vi "Test BMS communication.vi"() -> ()   [LabVIEW 2016]
uses:
  Program Files (x86)/National Instruments/LabVIEW 2016/examples/robotics/EPOS2 CANOpen Driver/Low Level VIs/Typedefs/FPGA CAN Frame Cluster.ctl
  Dashboard Control.ctl
  <vilib>/Utility/miscctls.llb/LVRowAndColumnUnsignedTypeDef.ctl
  <vilib>/Platform/TimedLoop/XDataNode/timing_clust.ctl
  <vilib>/Platform/TimedLoop/XDataNode/nitl_modes.ctl
  <vilib>/Platform/TimedLoop/XDataNode/wakeup.ctl
  RT/Read All CAN.vi
  <vilib>/Platform/TimedLoop/XDataNode/XDataNode.xnode
  <vilib>/Platform/TimedLoop/XDataNode/XDNodeRunTimeDep.lvlib
panel:
  in  "Tab Control":enum32{"Play!", "Debugg"}(tab)
  in  "Dashboard Control":T1 {"High Voltage" scale=0.0..255.0; "Low Voltage" scale=0.0..255.0}
  out "Tractive system activation":bool
  out "Ready to drive":bool
  in  "CAN Frame":T2={"Timestamp"=0, "Identifier"=0, "Type"=0, "InfoA"=0, "InfoB"=0, "DataLength"=0, "Data"=[0, 0, 0, 0, 0, 0, 0, 0]} {"Data" format="%.0x"; "DataLength" format="%.0x"; "InfoB" format="%.0x"; "InfoA" format="%.0x"; "Type" format="%.0x"; "Identifier" format="%.0x"; "Timestamp" format="%.0x"}
  in  "Send once":bool
  in  "Send cont.":bool
  in  "Stop":bool
  out "Error Out":errorcluster
  out "CAN Frame Out":T2 {"Data" format="%.0x"; "DataLength" format="%.0x"; "InfoB" format="%.0x"; "InfoA" format="%.0x"; "Type" format="%.0x"; "Identifier" format="%.0x"; "Timestamp" format="%.0x"}
  in  "Clear list":bool
  out "Multicolumn Listbox":i32(listbox)
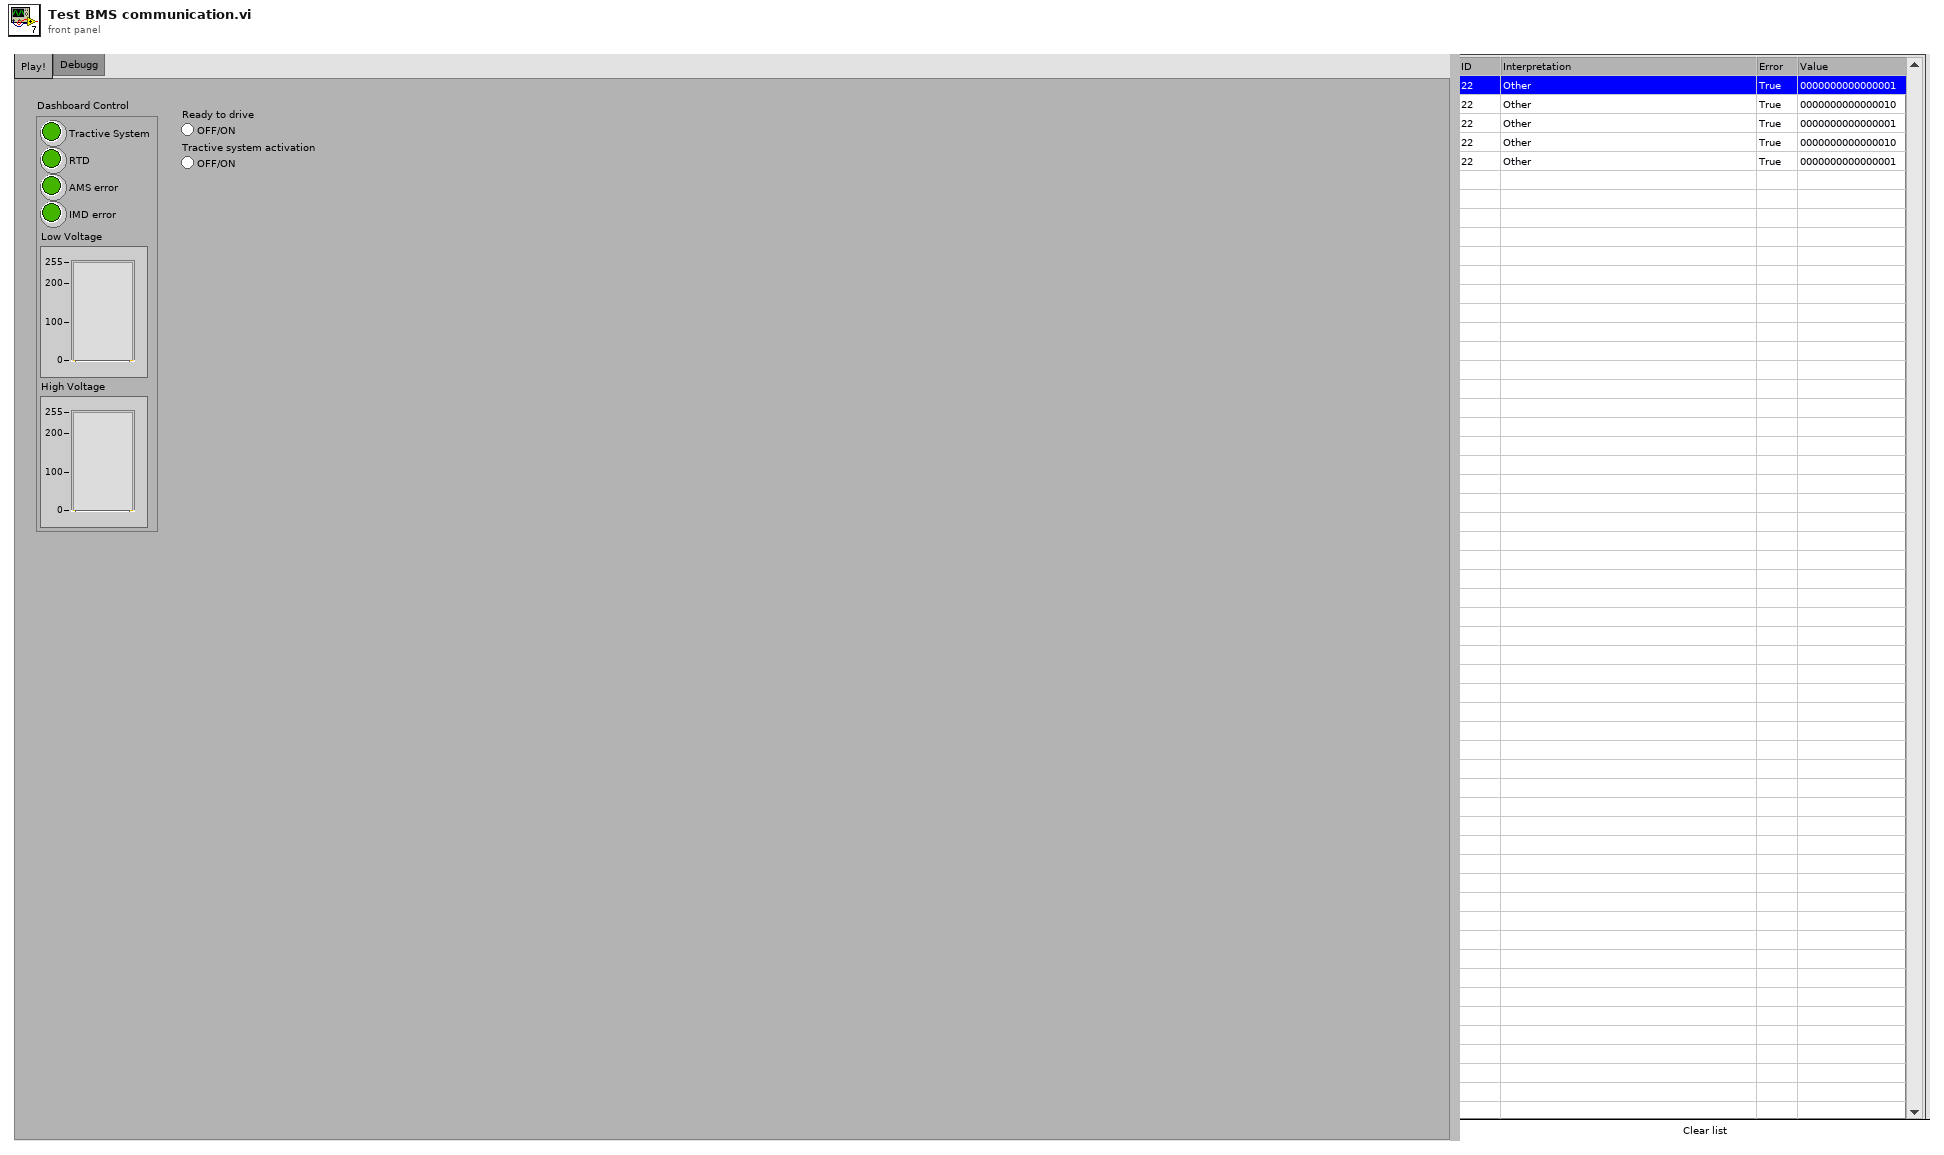
[diagram p1: front panel]
types:
  T1 = typedef "Dashboard Control.ctl" = cluster{"Tractive System":bool, "RTD":bool, "AMS error":bool, "IMD error":bool, "Low Voltage":dbl, "High Voltage":dbl}
  T2 = typedef "FPGA CAN Frame Cluster.ctl" = cluster{"Timestamp":u64, "Identifier":u32, "Type":u8, "InfoA":u8, "InfoB":u8, "DataLength":u8, "Data":u8[]}
  T3 = cluster{"Message":string, "ID":u16, "Error":bool}[]
  T4 = typedef "LVRowAndColumnUnsignedTypeDef.ctl" = cluster{"Row":u32, "Column":u32}
  T5 = typedef "XDNodeRunTimeDep.lvlib/timing_clust.ctl" = cluster{"Expected End [f-1]":u64, "Actual End [f-1]":u64, "Finished Late? [f-1]":bool, "Expected End [i-1]":u64, "Actual End [i-1]":u64, "Finished Late? [i-1]":bool, "Expected Start [i]":u64, "Actual Start [i]":u64, "Expected Start [f]":u64, "Actual Start [f]":u64, "Source Name":string, "Structure Name":string, "Period":i64, "Deadline":i64, "Offset":i64, "Start":i64, "Priority":i32, "Timeout":i32, "Mode":T6, "Wakeup Reason":T7, "Error":errorcluster, "Source Type":string, "Secondary Source Type":string, "Global End Time":u64, "Global Start Time":u64, "Frame Duration":u64, "Iteration Duration":u64, "Assigned CPU":i32, "I/O Scan Engine Mode":u32}
  T6 = typedef "XDNodeRunTimeDep.lvlib/nitl_modes.ctl" = enum32{"No Change", "Process missed periods, maintain original phase", "Discard missed periods, maintain original phase", "Process missed periods, ignore original phase", "Discard missed periods, ignore original phase"}
  T7 = typedef "XDNodeRunTimeDep.lvlib/wakeup.ctl" = enum32{"Normal", "Aborted", "Asynchronous wakeup", "Timing source error", "Timed loop error", "Timeout"}
  T8 = typedef "CAN Refnum.ctl" = refnum<k1>
  T9 = cluster{"Boolean array[0]":bool, "Boolean array[1]":bool, "Boolean array[2]":bool, "Boolean array[3]":bool, "Boolean array[4]":bool, "Boolean array[5]":bool, "Boolean array[6]":bool, "Boolean array[7]":bool, "Boolean array[8]":bool}
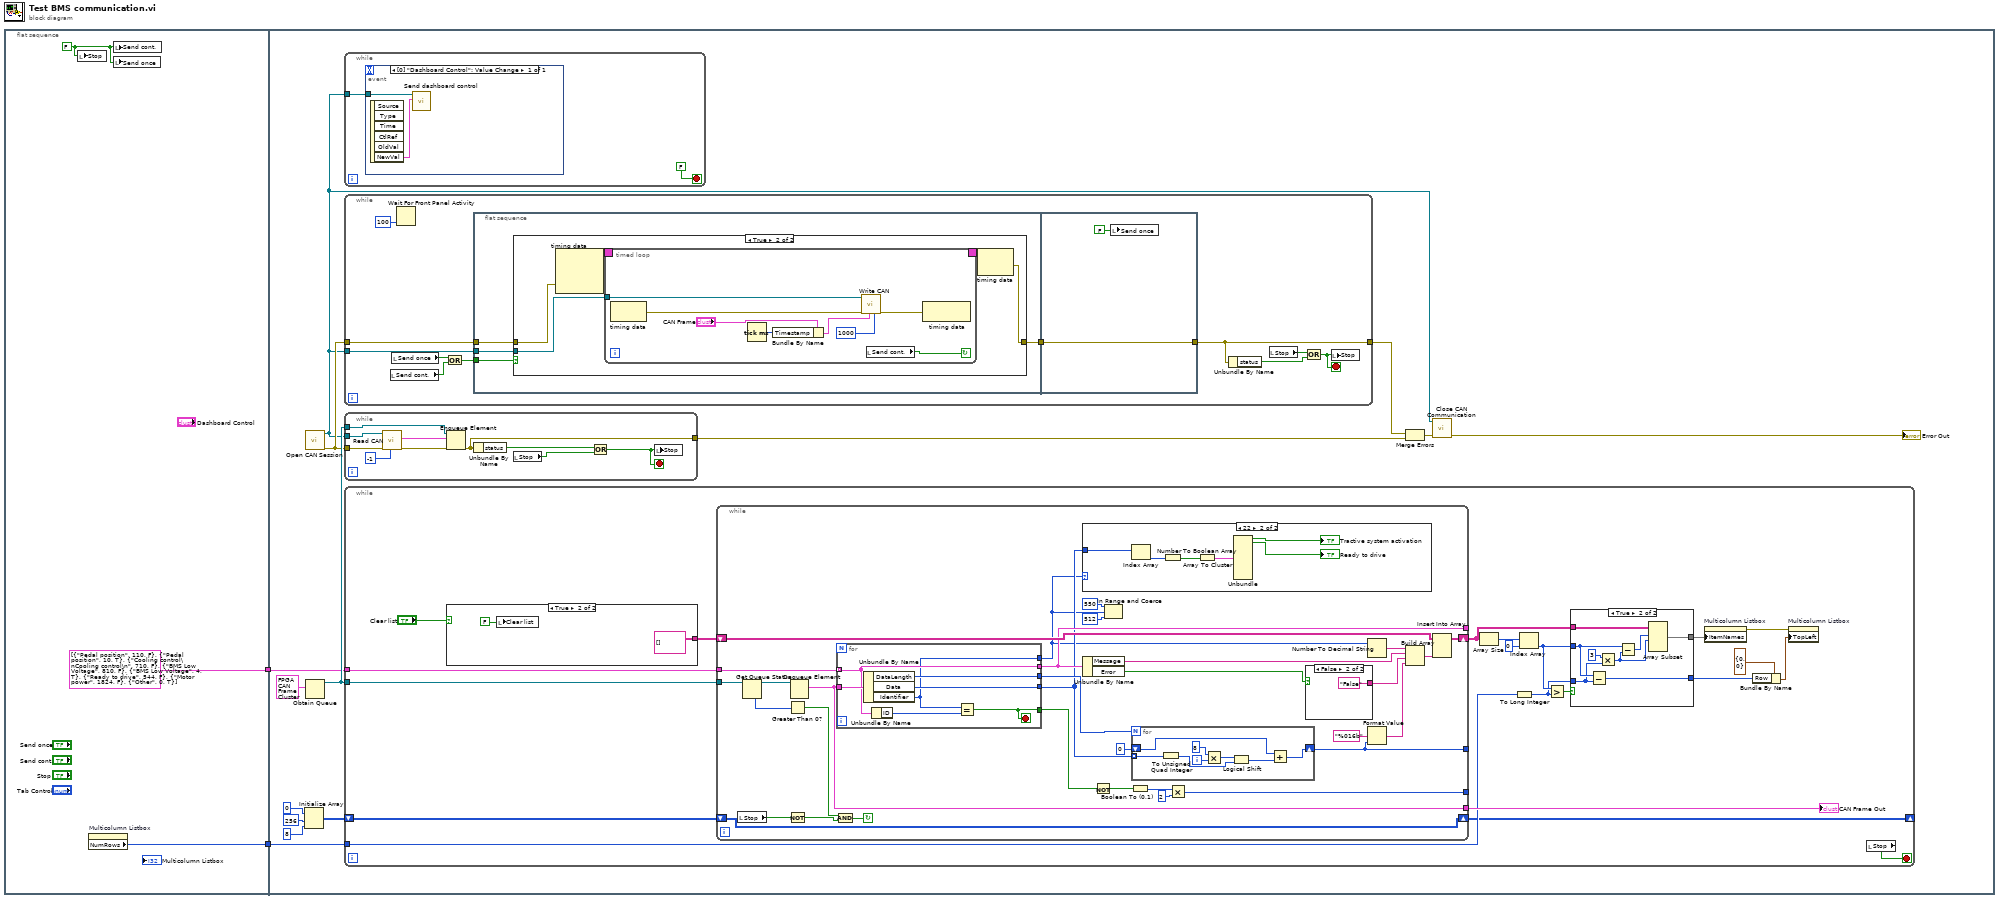
[diagram p0: block diagram]
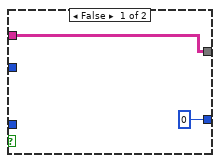
[diagram p2: hidden frame]
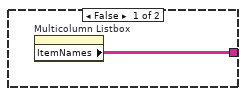
[diagram p3: hidden frame]
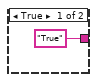
[diagram p5: hidden frame]
diagram:
  n1 = flat-sequence {
    tunnel: [w4] -> w2
    tunnel: [T3 [{"Message"="Pedal position", "ID"=110, "Error"=FALSE}, {"Message"="Pedal position", "ID"=10, "Error"=TRUE}, {"Message"="Cooling control\nCooling control\n", "ID"=710, "Error"=FALSE}, {"Message"="BMS Low Voltage", "ID"=810, "Error"=FALSE}, {"Message"="BMS Low Voltage", "ID"=4, "Error"=TRUE}, {"Message"="Ready to drive", "ID"=544, "Error"=FALSE}, {"Message"="Motor power", "ID"=1824, "Error"=FALSE}, {"Message"="Other", "ID"=0, "Error"=TRUE}] ("Messages")] -> w1
    tunnel: w2 -> [w14]
    tunnel: w1 -> [w13]
    frame #0 {
      w5 = FALSE
      n2 = local write "Stop"(w5) -> ()
      n3 = property on="Multicolumn Listbox" class="MCListbox (strict)"() -> ("NumRows"=w4:u32)  [unwired: 2 in, 2 out]
      n4 = local write "Send cont."(w5) -> ()
      n5 = local write "Send once"(w5) -> ()
    }
    frame #1 {
      n6 = Initialize Array(u8 0 ("element"), 256 ("dimension size"), 8 ("dimension size")) -> (w9:u8[][])
      n7 = call "Open CAN Session.vi"() -> ("error out"=w7:errorcluster, "CAN Session"=w6:T8)  [unwired: 10 in]
      n8 = Obtain Queue(element data type=T2 {"Timestamp"=0, "Identifier"=0, "Type"=0, "InfoA"=0, "InfoB"=0, "DataLength"=0, "Data"=[0, 0, 0, 0, 0, 0, 0, 0]} ("CAN Frame Out")) -> (queue out=w16:refnum<queue>)  [unwired: 4 in, 2 out]
      n9 = while {
        tunnel: w6 -> [w21]
        stop <- FALSE stop-if-true
        n10 = event shown="[0] \"Dashboard Control\": Value Change" {
          selector: _ -> [_]
          dyn-events: _ -> [_]
          timeout: _ -> [_]
          tunnel: w21 -> [w22]
          event Value Change {
            n11 = event-data() -> ("NewVal"=w23:T1)  [unwired: 1 in, 5 out]
            n12 = call "Send dashboard control.vi"("Dashboard Control"=w23, "CAN Session In"=w22) -> ()  [unwired: 8 in, 2 out]
          }
        }
      }
      n13 = while {
        tunnel: w7 -> [w132]
        tunnel: w6 -> [w131]
        tunnel: [w127] -> w18
        stop <- w123 stop-if-true
        n14 = local read "Send cont."() -> (w129:bool)
        n15 = local read "Send once"() -> (w128:bool)
        n16 = Wait For Front Panel Activity(1:100 ("timeout ms (-1 never timeout)")) -> ()  [unwired: 2 in, 1 out]
        n17 = Or(x=w128, y=w129) -> (x .or. y?=w130:bool)
        n18 = flat-sequence {
          tunnel: w132 -> [w136]
          tunnel: w131 -> [w135]
          tunnel: w130 -> [w134]
          tunnel: [w133] -> w122
          tunnel: [w162] -> w127
          tunnel: w122 -> [w162]
          frame #0 {
            n19 = case shown="True" w134 {
              tunnel: w136 -> [w137 w139]
              tunnel: w135 -> [_ w140]
              tunnel: [w137 w138] -> w133
              frame False {
              }
              frame True {
                n20 = node-c288(w139) -> (w142:T5)  [unwired: 2 in]
                n21 = timed-loop {
                  timing: w142 -> [_]
                  timing-out: [_] -> w141
                  tunnel: w140 -> [w150]
                  stop <- w147 continue-if-true
                  n22 = node-c288() -> (w149:errorcluster)  [unwired: 1 in]
                  n23 = Tick Count (ms)() -> (millisecond timer value=w143:u32)
                  n24 = Bundle By Name(cluster="CAN Frame", "Timestamp"=w143) -> (w144:T2)
                  n25 = call "Write CAN.vi"("timeout"=1000, "CAN Frame"=w144, "error in"=w149, "CAN Session In"=w150) -> ("error out"=w148:errorcluster)  [unwired: 6 in, 1 out]
                  n26 = local read "Send cont."() -> (w147:bool)
                  n27 = node-c288(w148) -> ()  [unwired: 1 out]
                }
                n28 = node-c288(w141) -> (w138:errorcluster)
              }
            }
          }
          frame #1 {
            n29 = local write "Send once"(FALSE) -> ()
          }
        }
        n30 = Unbundle By Name(w127) -> ("status"=w124:bool)
        n31 = local read "Stop"() -> (w125:bool)
        n32 = Or(x=w125, y=w124) -> (x .or. y?=w123:bool)
        n33 = local write "Stop"(w123) -> ()
      }
      n34 = while {
        tunnel: w7 -> [w113]
        tunnel: w6 -> [w112]
        tunnel: w16 -> [w119]
        tunnel: [w117] -> w15
        stop <- w120 stop-if-true
        n35 = call-poly "Read CAN.vi"("timeout in ms (-1)"=-1, "error in"=w113, "CAN Session In"=w112) -> ("error out"=w115:errorcluster, "CAN Frame Out"=w116:T2)  [unwired: 6 in, 1 out]
        n36 = Enqueue Element(queue=w119, element=w116, error in (no error)=w115) -> (error out=w117:errorcluster)  [unwired: 1 in, 2 out]
        n37 = Unbundle By Name(w117) -> ("status"=w118:bool)
        n38 = local read "Stop"() -> (w121:bool)
        n39 = Or(x=w118, y=w121) -> (x .or. y?=w120:bool)
        n40 = local write "Stop"(w120) -> ()
      }
      n41 = while {
        tunnel: w16 -> [w43]
        tunnel: w14 -> [w37]
        tunnel: w13 -> [w36]
        shift-right: [w24] -> _
        shift-left: w9 -> [w25]
        stop <- w41 stop-if-true
        n42 = case shown="True" "Clear list" {
          tunnel: [w54 string[][] [] ("Item Names")] -> w34
          frame False {
            n43 = property on="Multicolumn Listbox" class="MCListbox (strict)"() -> ("ItemNames"=w54:string[][])  [unwired: 2 in, 2 out]
          }
          frame True {
            n44 = local write "Clear list"(FALSE) -> ()
          }
        }
        n45 = while {
          tunnel: w43 -> [w86]
          tunnel: [w71] -> _
          tunnel: [w63] -> _
          tunnel: [w70] -> w42
          tunnel: [w69] -> _
          shift-right: [w72] -> w30
          shift-left: w34 -> [w73]
          tunnel: w36 -> [w68]
          shift-right: [w59] -> w24
          shift-left: w25 -> [w59]
          stop <- w64 continue-if-true
          n46 = local read "Stop"() -> (w67:bool)
          n47 = Get Queue Status(queue=w86) -> (queue out=w87:refnum<queue>, # elements in queue=w88:i32)  [unwired: 2 in, 6 out]
          n48 = Greater Than 0?(x=w88) -> (x > 0?=w65:bool)
          n49 = Not(x=w67) -> (.not. x?=w66:bool)
          n50 = Dequeue Element(queue=w87) -> (element=w70:T2)  [unwired: 2 in, 3 out]
          n51 = And(x=w65, y=w66) -> (x .and. y?=w64:bool)
          n52 = for {
            tunnel: w68 -> [w109] mode=indexing
            tunnel: w70 -> [w111]
            tunnel: [w109] -> w69
            tunnel: [w108] -> w75
            tunnel: [w107] -> w58
            tunnel: [w106] -> w74
            tunnel: [w105] -> w57
            stop <- w108 stop-if-true
            n53 = Unbundle By Name(w111) -> ("DataLength"=w106:u8, "Data"=w107:u8[], "Identifier"=w105:u32)
            n54 = Unbundle By Name(w109) -> ("ID"=w110:u16)
            n55 = Equal?(x=w105, y=w110) -> (x = y?=w108:bool)
          }
          n56 = case shown="22" w57 {
            tunnel: w58 -> [_ w93]
            frame 0, Default {
            }
            frame 22 {
              n57 = Index Array(array=w93) -> (element=w92:u8)  [unwired: 1 in]
              n58 = Number To Boolean Array(number=w92) -> (Boolean array=w91:bool[])
              n59 = Array To Cluster(array=w91) -> (cluster=w94:T9)
              n60 = Unbundle(w94) -> ("Boolean array[0]"=→"Tractive system activation":bool, "Boolean array[1]"=→"Ready to drive":bool)  [unwired: 7 out]
            }
          }
          n61 = Unbundle By Name(w69) -> ("Message"=w79:string, "Error"=w81:bool)
          n62 = Not(x=w75) -> (.not. x?=w78:bool)
          n63 = In Range and Coerce(upper limit=u16 550, x=w57, lower limit=u16 512) -> ()  [unwired: 2 out]
          n64 = Boolean To (0,1)(Boolean=w78) -> (0, 1=w76:i16)
          n65 = for {
            N: w74 -> [_]
            shift-right: [w96] -> w63
            shift-left: u64 0 -> [w98]
            tunnel: w58 -> [w95] mode=indexing
            i -> [w100]
            n66 = To Unsigned Quad Integer(1:w95) -> (0:w97:u64)
            n67 = Multiply(x=i8 8, y=w100) -> (x*y=w99:i32)
            n68 = Logical Shift(y=w99, x=w97) -> (x << y=w102:u64)
            n69 = Add(x=w98, y=w102) -> (x+y=w96:u64)
          }
          n70 = Multiply(x=w76, y=i16 2) -> (x*y=w71:i16)
          n71 = case shown="False" w81 {
            tunnel: ["True" "False"] -> w82
            frame True {
            }
            frame False {
            }
          }
          n72 = Number To Decimal String(number=w57) -> (decimal integer string=w80:string)  [unwired: 1 in]
          n73 = Format Value(format string="%016b", value (0)=w63) -> (output string=w84:string)  [unwired: 1 in]
          n74 = Build Array(w80, w79, w82, w84) -> (w83:string[])
          n75 = Insert Into Array(array=w73, new element=w83) -> (w72:string[][])  [unwired: 2 in]
        }
        "CAN Frame Out" <- w42
        n76 = Array Size(array=w30) -> (size(s)=w32:i32[])
        n77 = To Long Integer(number=w37) -> (32bit integer=w27:i32)
        n78 = Index Array(array=w32, index=0) -> (element=w28:i32)
        n79 = Greater?(x=w28, y=w27) -> (0:w26:bool)
        n80 = case shown="True" w26 {
          tunnel: [0 w46] -> w31
          tunnel: w27 -> [_ w47]
          tunnel: w28 -> [_ w48]
          tunnel: w30 -> [w44 w51]
          tunnel: [w44 w50] -> w29
          frame False {
          }
          frame True {
            n81 = Subtract(x=w48, y=w47) -> (x-y=w46:i32)
            n82 = Multiply(x=3, y=w47) -> (x*y=w52:i32)
            n83 = Subtract(x=w48, y=w52) -> (x-y=w53:i32)
            n84 = Array Subset(array=w51, index (row)=w53, length (row)=w52) -> (w50:string[][])  [unwired: 2 in]
          }
        }
        n85 = property on="Multicolumn Listbox" class="MCListbox (strict)"("ItemNames"=w29) -> (error out=w33:errorcluster)  [unwired: 2 in, 1 out]
        n86 = Bundle By Name(cluster=T4 {"Row"=0, "Column"=0} ("Top Left Visible Cell"), "Row"=w31) -> (w40:T4)
        n87 = property on="Multicolumn Listbox" class="MCListbox (strict)"(error in=w33, "TopLeft"=w40) -> ()  [unwired: 1 in, 2 out]
        n88 = local read "Stop"() -> (w41:bool)
      }
      n89 = Merge Errors(w18, w15) -> (w19:errorcluster)
      n90 = call "Close CAN Communication.vi"("error in"=w19, "CAN Session"=w6) -> ("error out"=→"Error Out":errorcluster)  [unwired: 9 in]
    }
  }
